vi "Scan Send Data Command Response.vi"(0 "Measurements In":dbl[](array[numeric]), 1 "Sensor Response":string, 2 "Total Measurements In":i32, 3 "Expected Measurements (1)":i32=1, 4 "Measurement Type In (Normal)":i32(ring) items=["Normal", "Concurrent", "Continuous"], 5 "Error In (No Error)":errorcluster, 6 "CRC (False)":bool, 7 "Parameter In (0)":i32(ring) items=["0", "1", "2", "3", "4", "5", "6", "7", "8", "9"], 10 "Sensor Address In":string="a") -> (14 "Measurements Out":dbl[](array[numeric]), 16 "Total Measurements Out":i32, 17 "Complete?":bool, 18 "CRC Message Out":string, 19 "Error Out":errorcluster)   [LabVIEW 2016, in "SDI-12.lvlib"]
doc: "Scans a sensor's response to one of the Send Data Command messages. Extracts and returns the Measurements contained within the sensor's message. If any Measurements are contained within the corresponding Measurements input, the new ones will be appended to those before being returned to the calling VI. This VI also keeps track of how many messages have been obtained from this sensor read in total, and if it is provided with the Expected Measurements input, it will flag the output boolean \"Complete?\" indicating that no further Send Data commands are needed for the current Read.\n\nRecall that each single Read with a sensor could contain up to 10 exchanges between the datalogger and the Sensor, and up to 20 measurement data points."
uses:
  SDI-12.lvlib
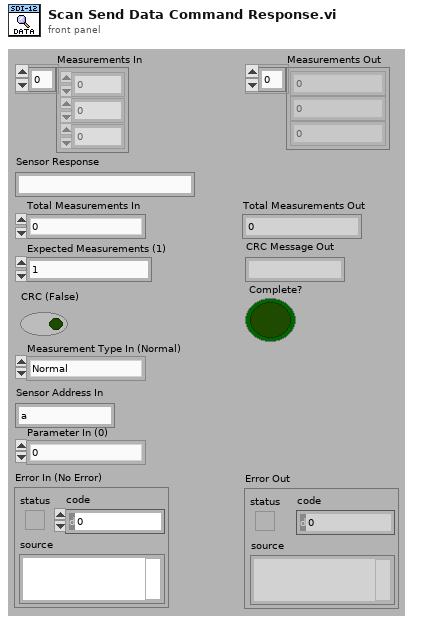
[diagram p1: front panel]
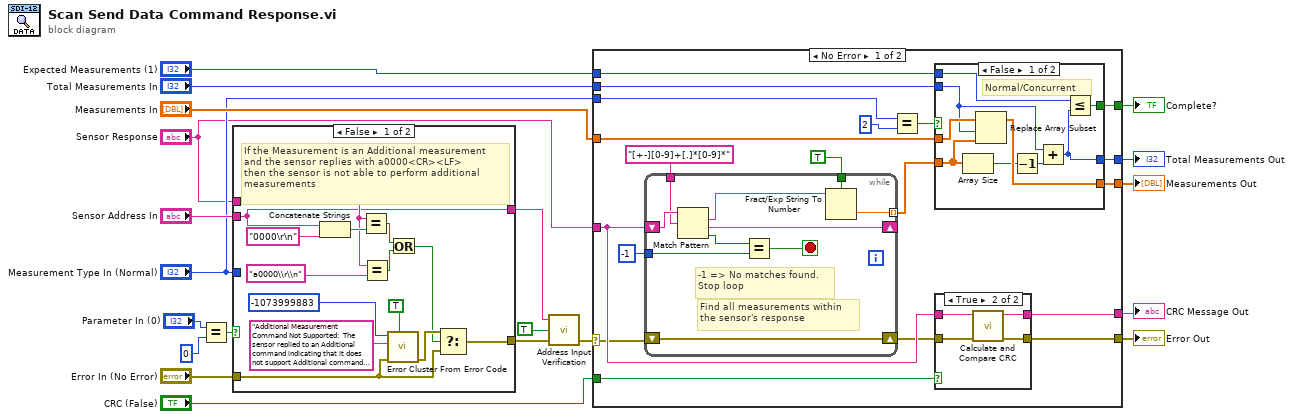
[diagram p0: block diagram]
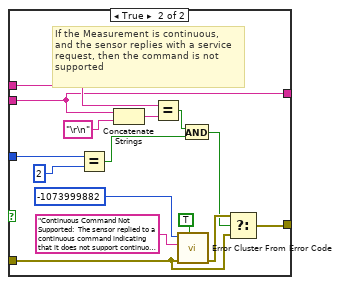
[diagram p2: hidden frame]
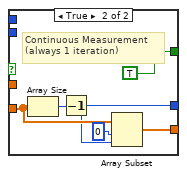
[diagram p3: hidden frame]
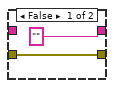
[diagram p4: hidden frame]
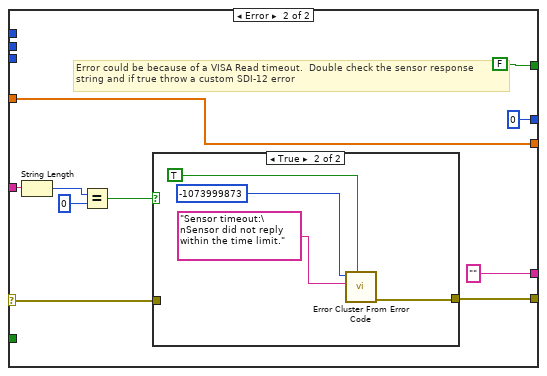
[diagram p5: hidden frame]
diagram:
  n1 = Equal?(x="Parameter In (0)", y=0) -> (x = y?=w5:bool)
  n2 = case shown="False" w5 {
    tunnel: [w27 w49] -> w12
    tunnel: "Error In (No Error)" -> [w28 w48]
    tunnel: "Measurement Type In (Normal)" -> [_ w47]
    tunnel: "Sensor Address In" -> [w21 w35]
    tunnel: "Sensor Response" -> [w23 w36]
    tunnel: [w21 w35] -> w1
    frame False {
      # "If the Measurement is an Additional measurement\nand the sensor replies with a0000<CR><LF>\nthen the sensor is not able to perform additional\nmeasurements"
      n3 = Concatenate Strings(w21, "0000\r\n") -> (w33:string)
      n4 = Equal?(x=w23, y=w33) -> (x = y?=w26:bool)
      n5 = Equal?(x=w23, y="a0000\\r\\n" ("read buffer")) -> (x = y?=w25:bool)
      n6 = call <vilib>:"Error Cluster From Error Code.vi"("show call chain? (False)"=TRUE, "error in (no error)"=w28, "error message (\"\")"="Additional Measurement Command Not Supported:  The sensor replied to an Additional command indicating that it does not support Additional commands for the current Measurement Type.  Your sensor may support Additional for a different type." ("error message (\"\")"), "error code (0)"=-1073999883 ("error code")) -> ("error out"=w29:errorcluster)  [unwired: 5 in]
      n7 = Or(x=w26, y=w25) -> (x .or. y?=w22:bool)
      n8 = Select(t=w29, s=w22, f=w28) -> (s? t:f=w27:errorcluster)
    }
    frame True {
      # "If the Measurement is continuous,\nand the sensor replies with a service\nrequest, then the command is not \nsupported"
      n9 = Equal?(x=w47, y=2) -> (x = y?=w44:bool)
      n10 = Concatenate Strings(w35, "\r\n") -> (w42:string)
      n11 = Equal?(x=w36, y=w42) -> (x = y?=w45:bool)
      n12 = call <vilib>:"Error Cluster From Error Code.vi"("show call chain? (False)"=TRUE, "error in (no error)"=w48, "error message (\"\")"="Continuous Command Not Supported:  The sensor replied to a continuous command indicating that it does not support continuous commands." ("error message (\"\")"), "error code (0)"=-1073999882 ("error code")) -> ("error out"=w38:errorcluster)  [unwired: 5 in]
      n13 = And(x=w45, y=w44) -> (x .and. y?=w37:bool)
      n14 = Select(t=w38, s=w37, f=w48) -> (s? t:f=w49:errorcluster)
    }
  }
  n15 = call "Address Input Verification.vi"("Error In (No Error)"=w12, "Error if Bad? (True)"=TRUE ("error if bad? (True)"), "Sensor Address In (a)"=w1) -> ("Error Out"=w19:errorcluster)  [unwired: 1 in, 1 out]
  n16 = case shown="No Error" w19 {
    selector: w19 -> [w65 w104]
    tunnel: "Sensor Response" -> [w68 w109]
    tunnel: [w66 w105] -> w20
    tunnel: [w64 "" ("sent CRC")] -> w18
    tunnel: [w55 FALSE] -> w17
    tunnel: [w53 0] -> w16
    tunnel: [w57 w100] -> w15
    tunnel: "Measurements In" -> [w59 w100]
    tunnel: "Expected Measurements (1)" -> [w54 _]
    tunnel: "CRC (False)" -> [w60 _]
    tunnel: "Total Measurements In" -> [w56 _]
    tunnel: "Measurement Type In (Normal)" -> [w50 _]
    frame No Error {
      n17 = while {
        shift-right: [w90] -> _
        shift-left: w68 -> [w97]
        shift-right: [w99] -> w67
        shift-left: w65 -> [w99]
        tunnel: [w98] -> w58 mode=indexing
        tunnel: "[+-][0-9]+[.]*[0-9]*" ("regular expression") -> [w94]
        tunnel: -1 ("y") -> [w93]
        tunnel: TRUE ("use system decimal point (T)") -> [w92]
        stop <- w95 stop-if-true
        # "Find all measurements within \nthe sensor's response"
        # "-1 => No matches found.\nStop loop"
        n18 = Match Pattern(string=w97, regular expression=w94) -> (match substring=w91:string, after substring=w90:string, offset past match=w96:i32)  [unwired: 1 in, 1 out]
        n19 = Equal?(x=w96, y=w93) -> (x = y?=w95:bool)
        n20 = Fract/Exp String To Number(use system decimal point (T)=w92, string=w91) -> (number=w98:dbl)  [unwired: 2 in, 1 out]
      }
      n21 = Equal?(x=w50, y=2) -> (x = y?=w52:bool)
      n22 = case shown="False" w52 {
        tunnel: w59 -> [w77 _]
        tunnel: w58 -> [w73 w81]
        tunnel: [w76 w78] -> w57
        tunnel: w56 -> [w72 _]
        tunnel: [w75 TRUE] -> w55
        tunnel: w54 -> [w74 _]
        tunnel: [w69 w80] -> w53
        frame False {
          # "Normal/Concurrent"
          n23 = Array Size(array=w73) -> (size(s)=w71:i32)
          n24 = Replace Array Subset(array=w77, new element=w73, index=w72) -> (w76:dbl[])
          n25 = Decrement(x=w71) -> (x-1=w70:i32)
          n26 = Add(x=w72, y=w70) -> (x+y=w69:i32)
          n27 = Less Or Equal?(x=w74, y=w69) -> (x <= y?=w75:bool)
        }
        frame True {
          # "Continuous Measurement\n(always 1 iteration)"
          n28 = Array Size(array=w81) -> (size(s)=w82:i32)
          n29 = Decrement(x=w82) -> (x-1=w80:i32)
          n30 = Array Subset(array=w81, index=0, length=w80) -> (w78:dbl[])
        }
      }
      n31 = case shown="True" w60 {
        tunnel: [w84 w89] -> w66
        tunnel: ["" ("sent CRC") w88] -> w64
        tunnel: w67 -> [w84 w87]
        tunnel: w68 -> [_ w86]
        frame False {
        }
        frame True {
          n32 = call "Calculate and Compare CRC.vi"("Error In (No Error)"=w87, "Sensor Response"=w86) -> ("Error Out"=w89:errorcluster, "Sent CRC"=w88:string)  [unwired: 6 in, 2 out]
        }
      }
    }
    frame Error {
      # "Error could be because of a VISA Read timeout.  Double check the sensor response\nstring and if true throw a custom SDI-12 error"
      n33 = String Length(string=w109) -> (length=w108:i32)
      n34 = Equal?(x=w108, y=0) -> (x = y?=w107:bool)
      n35 = case shown="True" w107 {
        tunnel: [w110 w112] -> w105
        tunnel: w104 -> [w110 _]
        frame False {
        }
        frame True {
          n36 = call <vilib>:"Error Cluster From Error Code.vi"("show call chain? (False)"=TRUE, "error message (\"\")"="Sensor timeout:\nSensor did not reply within the time limit." ("error message (\"\")"), "error code (0)"=-1073999873 ("error code")) -> ("error out"=w112:errorcluster)  [unwired: 6 in]
        }
      }
    }
  }
  "Error Out" <- w20
  "CRC Message Out" <- w18
  "Total Measurements Out" <- w16
  "Complete?" <- w17
  "Measurements Out" <- w15
